vi "CalculatePerpendicularLine2.vi"(10 "Start":cluster{"X":dbl, "Y":dbl}, 11 "Cluster in":T1) -> (3 "Cluster out":T2)   [LabVIEW 2019]
uses:
  <vilib>/vision/NI_Vision_Development_Module.lvlib
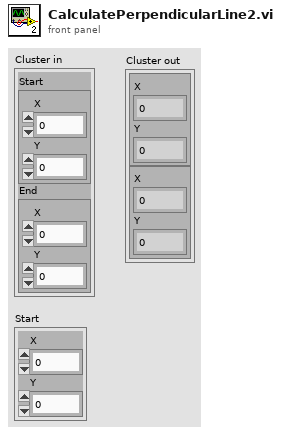
[diagram p1: front panel]
types:
  T1 = cluster{"Start":cluster{"X":dbl, "Y":dbl}, "End":cluster{"X":dbl, "Y":dbl}}
  T2 = cluster{cluster{"X":dbl, "Y":dbl}, cluster{"X":dbl, "Y":dbl}}
  T3 = cluster{"Point 1":cluster{"X":sgl, "Y":sgl}, "Point 2":cluster{"X":sgl, "Y":sgl}}
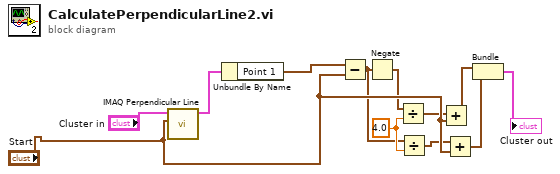
[diagram p0: block diagram]
diagram:
  w7 = 4.0
  n1 = call "IMAQ Perpendicular Line"("Point"="Start", "Line"="Cluster in") -> ("Perpendicular Line"=w2:T3)  [unwired: 7 in, 2 out]
  n2 = Unbundle By Name(w2) -> ("Point 1"=w3:cluster{"X":sgl, "Y":sgl})
  n3 = Subtract(x=w3, y="Start") -> (x-y=w6:cluster{"X":dbl, "Y":dbl})
  n4 = Negate(x=w6) -> (-x=w5:cluster{"X":dbl, "Y":dbl})
  n5 = Divide(x=w5, y=w7) -> (x/y=w8:cluster{"X":dbl, "Y":dbl})
  n6 = Divide(x=w6, y=w7) -> (x/y=w10:cluster{"X":dbl, "Y":dbl})
  n7 = Add(x=w8, y="Start") -> (x+y=w9:cluster{"X":dbl, "Y":dbl})
  n8 = Add(x=w10, y="Start") -> (x+y=w12:cluster{"X":dbl, "Y":dbl})
  n9 = Bundle(w9, w12) -> (→"Cluster out":T2)  [unwired: 1 in]
